vi "Date Setup.vi"(0 "VISA resource name":refnum<visa-resource-name>, 1 "Hour":i16=1 min=1 max=31, 2 "Minute":i16=1 min=1 max=31, 3 "Second":i16=1 min=1 max=31, 5 "Date":i16=31 min=1 max=31, 7 "Month":i16=12 min=1 max=12, 9 "Year":i16=2001 min=2000 max=2099, 11 "error in (no error)":errorcluster, 12 "Mode (T: Manual)":bool=TRUE) -> (4 "VISA resource name out":refnum<visa-resource-name>, 15 "error out":errorcluster)   [LabVIEW 2013, in "LeCroy Wave Series.lvlib"]
doc: "The instrument gives you the choice of manually setting the time and date or getting it from the Internet. If you select to get the time and date from the Internet, you need to have the scope connected to the Internet through the LAN connector on the rear panel."
uses:
  LeCroy Wave Series.lvlib
panel:
  # "Manual\n\nFrom Internet"
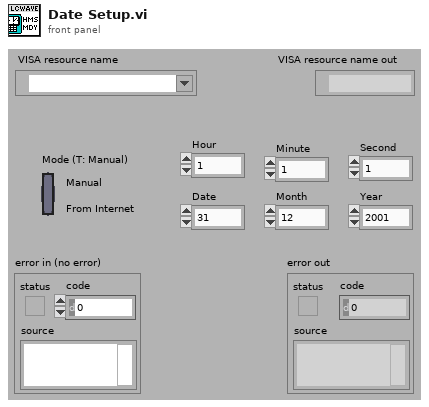
[diagram p1: front panel]
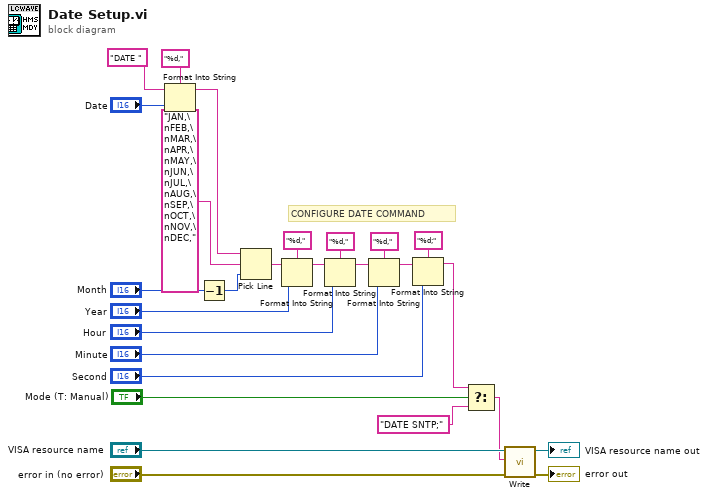
[diagram p0: block diagram]
diagram:
  # "CONFIGURE DATE COMMAND"
  n1 = Format Into String(format string="%d,", initial string="DATE ", "Date") -> (resulting string=w17:string)  [unwired: 1 in, 1 out]
  n2 = Decrement(x="Month") -> (x-1=w22:i16)
  n3 = Pick Line(string ("")=w17, multi-line string="JAN,\nFEB,\nMAR,\nAPR,\nMAY,\nJUN,\nJUL,\nAUG,\nSEP,\nOCT,\nNOV,\nDEC,", line index=w22) -> (output string=w16:string)
  n4 = Format Into String(format string="%d,", initial string=w16, "Year") -> (resulting string=w12:string)  [unwired: 1 in, 1 out]
  n5 = Format Into String(format string="%d,", initial string=w12, "Hour") -> (resulting string=w9:string)  [unwired: 1 in, 1 out]
  n6 = Format Into String(format string="%d,", initial string=w9, "Minute") -> (resulting string=w5:string)  [unwired: 1 in, 1 out]
  n7 = Format Into String(format string="%d;", initial string=w5, "Second") -> (resulting string=w4:string)  [unwired: 1 in, 1 out]
  n8 = Select(t=w4, s="Mode (T: Manual)", f="DATE SNTP;") -> (s? t:f=w1:string)
  n9 = call "Write.vi"("error in (no error)"="error in (no error)", "Write Buffer"=w1, "VISA resource name"="VISA resource name") -> ("error out"=→"error out":errorcluster, "VISA resource name out"=→"VISA resource name out":refnum<visa-resource-name>)  [unwired: 6 in, 1 out]
